vi "Dashboard Main.vi"() -> ()   [LabVIEW 2013]
uses:
  <vilib>/event_ctls.llb/eventvkey.ctl
  <vilib>/Rock Robotics/WPI/Dashboard/WPI_DashboardLogging Global.vi
  <vilib>/Utility/config.llb/Write Key (String).vi
  <vilib>/Utility/config.llb/Write Key (I32).vi
  <vilib>/Utility/config.llb/NI_LVConfig.lvlib
panel:
  out "Image Message":string="Timeout in Camera Communications"
  in  "Rec Mode":enum32{"Stop", "Record", "Playback"}(radio)
  in  "Dashboard Tab":T1(tab)=enum."Auto"
  in  "Camera Settings":T2={"Frame Rate"=30, "Compression"=30, "Size"=1} {"Frame Rate" scale=1.0..30.0; "Size" items=["640x480", "320x240", "160x120"]}
  out "MotorSliders R":cluster{"MotorSlide1":dbl, "MotorSlide2":dbl} {"MotorSlide2" scale=-1.0..1.0 scale format="%#_2e"; "MotorSlide1" scale=-1.0..1.0 scale format="%#_2e"}
  out "MotorChart R":cluster{"Numeric":dbl, "Numeric":dbl}(graph)
  out "MotorSliders L":T3 {"MotorSlide4 2" scale=0.0..14.0 scale format="%#_2e"; "MotorSlide2" scale=-1.0..1.0 scale format="%#_2e"; "MotorSlide1" scale=-1.0..1.0 scale format="%#_2e"}
  out "MotorChart L":T4(graph)
  out "JS1 Z":dbl(slide) scale=-1.0..1.0 scale format="%#_2e"
  out "Joystick 1":cluster{"X":dbl, "Y":dbl}[](graph)
  out "JS Buttons 1":T5
  out "JS2 Z":dbl(slide) scale=-1.0..1.0 scale format="%#_2e"
  out "Joystick 2":cluster{"X":dbl, "Y":dbl}[](graph)
  out "JS Buttons 2":T5
  out "Mode":T6(ring)=enum."Auto Disabled"
  out "Camera IP":string
  in  "DB Camera Config":bool
  out "fps":dbl format="%#.1g"
  out "Mbps":dbl format="%#.1g"
  out "Mbps 2":bool
  out "LED 1":bool
  in  "Slider 1":dbl(slide) scale=0.0..100.0
  in  "Auton Selection":dbl=5.0
  out "key":T7(ring)
  in  "Checkbox 2":bool
  in  "Checkbox 1":bool
  out "Code":dbl
  in  "Test Slider":dbl(slide) scale=0.0..100.0 scale format="%#_3g"
  in  "On/Off":bool caption="Solenoid"
  in  "Test Name":u16(ring) items=["Select the test to run...", "Example Test", "-------------------------------", "List of tests is built in robot code.", "Replace with your own automated tests."]
  in  "Test Tree":string(tree)
  in  "Motor":cluster{"Value":dbl, "Enable":bool} {"Value" scale=-1.0..1.0 scale format="%#_3g"}
  out "Progress":T8 {"Test Progress" scale=0.0..100.0}
  in  "Rev/Fwd":cluster{"Forward":bool, "Reverse":bool}
  in  "Test Ring":u16(ring) items=["Auto", "Fixed indoor", "Fixed outdoor 1", "Fixed outdoor 2", "Fixed fluorescent 1", "Fixed fluorescent 2", "Hold current"]
  in  "Listbox":i32(listbox)
  out "Tree":string(tree)
  out "Camera Image":T9(plugin-control)
  in  "Enable":bool
  # "Left"
  # "Front"
  # "Right"
  # "Battery"
  # "Customize by placing controls and indicators here and name to\nmatch Dashboard Variables on robot."
  # "This tab is a great place for autonomous settings and validation.\nCustomize by placing controls and indicators here and name to\nmatch Dashboard Variables on robot."
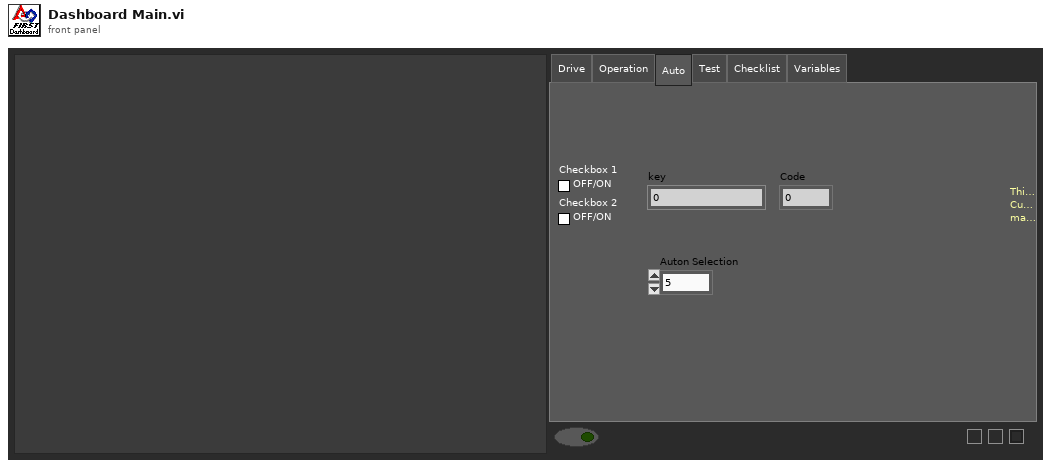
[diagram p1: front panel]
types:
  T1 = enum32{"Drive", "Operation", "Auto", "Test", "Checklist", "Variables"}
  T2 = cluster{"Frame Rate":i32, "Compression":i32, "Size":u16}
  T3 = cluster{"MotorSlide1":dbl, "MotorSlide2":dbl, "MotorSlide4 2":dbl}
  T4 = cluster{"Numeric":dbl, "Numeric":dbl, "Battery":sgl}
  T5 = cluster{bool, bool, bool, bool, bool, bool, bool, bool, bool, bool, bool, bool}
  T6 = enum8{"Tele-Op Disabled", "Tele-Op Enabled", "Auto Disabled", "Auto Enabled", "Test Disabled", "Test Enabled", ""}
  T7 = enum16{"0", "1", "2", "3", "4", "5", "6", "7", "8", "9", "A", "B", "C", "D", "E", "F", "G", "H", "I", "J", "K", "L", "M", "N", "O", "P", "Q", "R", "S", "T", "U", "V", "W", "X", "Y", "Z", "F1", "F2", "F3", "F4", "F5", "F6", "F7", "F8", "F9", "F10", "F11", "F12", "F13", "F14", "F15", "ADD", "BACK", "BACKSLASH", "CAPITAL", "COMMA", "DECIMAL", "DELETE", "DIVIDE", "DOWN", "END", "EQUALS", "ESCAPE", "GRAVE (`)", "HOME", "INSERT", "LBRACKET", "LCONTROL", "LEFT", "L ALT", "LSHIFT", "LWIN", "MINUS", "MULTIPLY", "NEXT", "NUMLOCK", "NUMPAD_0", "NUMPAD_1", "NUMPAD_2", "NUMPAD_3", "NUMPAD_4", "NUMPAD_5", "NUMPAD_6", "NUMPAD_7", "NUMPAD_8", "NUMPAD_9", "PAUSE", "PERIOD", "PRIOR (PG UP)", "RBRACKET", "RCONTROL", "RETURN", "RIGHT", "R ALT", "RSHIFT", "RWIN", "SCROLL", "SEMICOLON", "SLASH", "SPACE", "SUBTRACT", "TAB", "UP", "ENTER (num pad)", "' (quote)"}
  T8 = cluster{"Test Progress":u8, "Test Progress Text":string}
  T9 = typedef "IMAQ Image.ctl" = refnum<image>
  T10 = typedef "Image Type" = u32
  T11 = cluster{"Digital Inputs":bool[], "Digital Outputs":bool[]}
  T12 = cluster{"Competition mode":bool, "Robot Link":bool, "Autonomous":bool, "Enabled":bool, "E-Stop":bool, "Simulated":bool, "TestMode":bool, "Docked Window":bool}
  T13 = cluster{"Boolean Array[0]":bool, "Boolean Array[1]":bool, "Boolean Array[2]":bool, "Boolean Array[3]":bool, "Boolean Array[4]":bool, "Boolean Array[5]":bool, "Boolean Array[6]":bool, "Boolean Array[7]":bool, "Boolean Array[8]":bool, "Boolean Array[9]":bool, "Boolean Array[10]":bool, "Boolean Array[11]":bool}
  T14 = typedef "NI_LVConfig.lvlib/Config Data RefNum.ctl" = refnum<k1>
  T15 = typedef "eventvkey.ctl" = enum16{"ASCII", "Enter", "Return", "Shift", "Ctrl", "Alt", "Cmd", "Opt", "Caps", "NumLock", "Clear", "Break", "Up", "Down", "Left", "Right", "Insert", "Delete", "Home", "End", "PageUp", "PageDown", "Escape", "Help", "Pause", "ScrollLock", "F1", "F2", "F3", "F4", "F5", "F6", "F7", "F8", "F9", "F10", "F11", "F12", "F13", "F14", "F15", "F16", "F17", "F18", "F19", "F20", "F21", "F22", "F23", "F24", "Play", "VolumeUp", "VolumeDown", "Mute", "Two Byte Char"}
  T16 = cluster{"Image Size":bool, "Image Type":bool, "Pixel Value":bool, "ROI Information":bool, "Zoom Factor":bool}
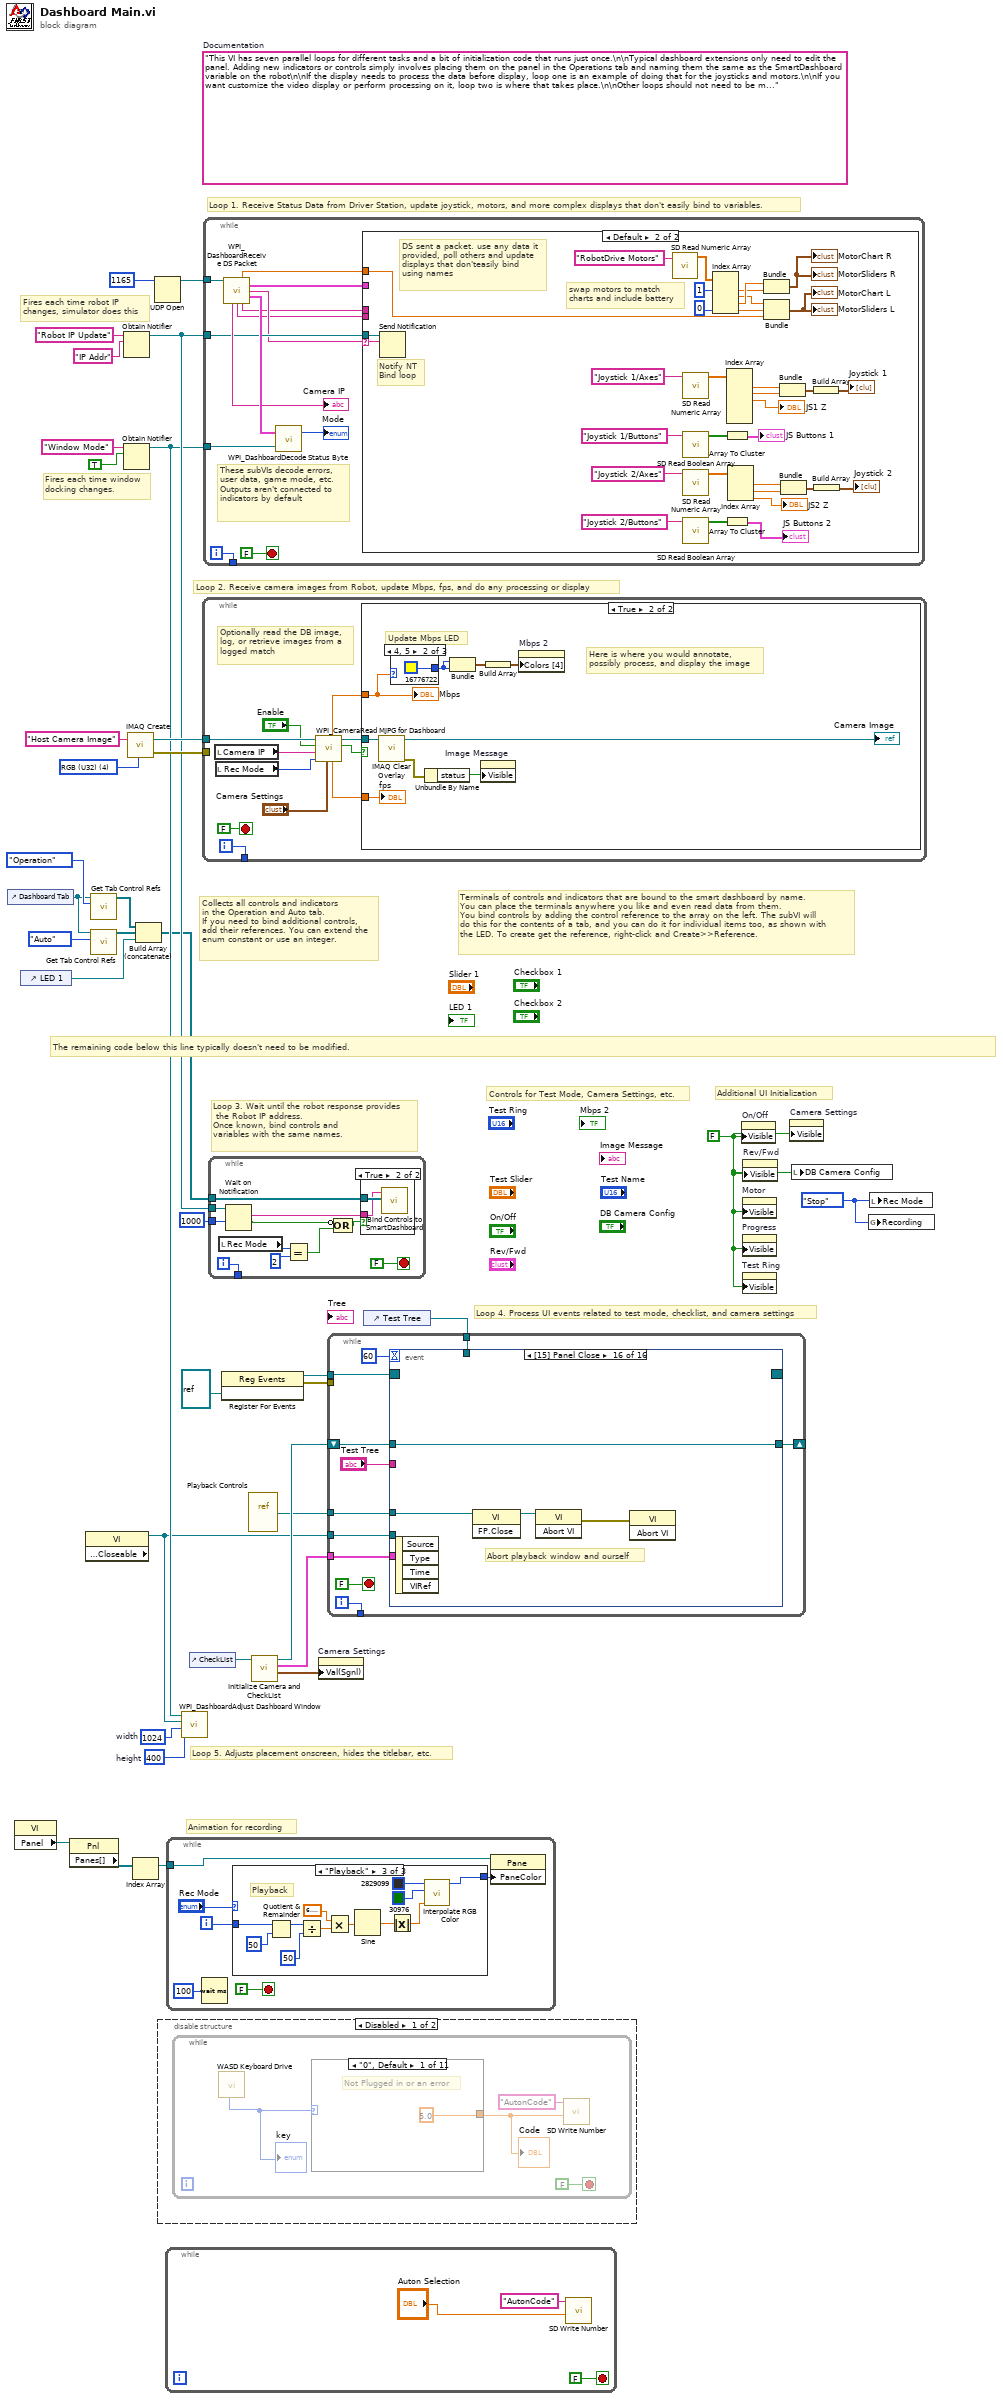
[diagram p0: block diagram]
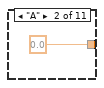
[diagram p2: hidden frame]
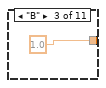
[diagram p3: hidden frame]
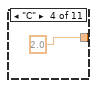
[diagram p4: hidden frame]
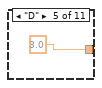
[diagram p5: hidden frame]
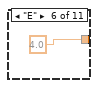
[diagram p6: hidden frame]
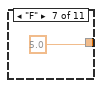
[diagram p7: hidden frame]
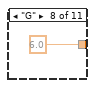
[diagram p8: hidden frame]
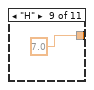
[diagram p9: hidden frame]
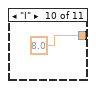
[diagram p10: hidden frame]
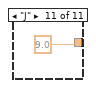
[diagram p11: hidden frame]
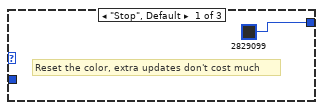
[diagram p13: hidden frame]
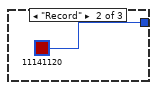
[diagram p14: hidden frame]
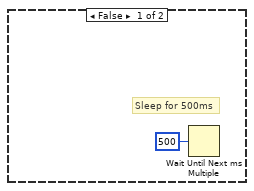
[diagram p16: hidden frame]
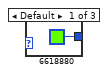
[diagram p17: hidden frame]
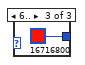
[diagram p18: hidden frame]
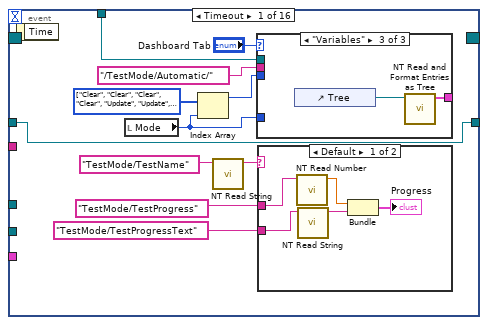
[diagram p19: hidden frame]
diagram:
  w8 = enum32{"Stop", "Record", "Playback"}."Stop" ("Rec Mode")
  w11 = 400  # height
  w12 = 1024  # width
  w25 = FALSE ("Visible")
  (unwired) "This VI has seven parallel loops for different tasks and a bit of initialization code that runs just once.\n\nTypical dashboard extensions only need to edit the panel. Adding new indicators or controls simply involves placing them on the panel in the Operations tab and naming them the same as the SmartDashboard variable on the robot\n\nIf the display needs to process the data before display, loop one is an example of doing that for the joysticks and motors.\n\nIf you want customize the video display or perform processing on it, loop two is where that takes place.\n\nOther loops should not need to be modified. They are pretty standard, and document the task they perform."  # Documentation
  w35 = T10 4 items=["Grayscale (U8)", "Grayscale (I16)", "Grayscale (SGL)", "Complex (CSG)", "RGB (U32)", "HSL (U32)", "RGB (U64)"] ("Image Type")
  # "Controls for Test Mode, Camera Settings, etc."
  # "Additional UI Initialization"
  # "Animation for recording"
  # "Fires each time robot IP\nchanges, simulator does this"
  # "Fires each time window\ndocking changes."
  # "Collects all controls and indicators\nin the Operation and Auto tab.\nIf you need to bind additional controls,\nadd their references. You can extend the\nenum constant or use an integer."
  # "The remaining code below this line typically doesn't need to be modified."
  # "Loop 4. Process UI events related to test mode, checklist, and camera settings"
  # "Terminals of controls and indicators that are bound to the smart dashboard by name.\nYou can place the terminals anywhere you like and even read data from them.\nYou bind controls by adding the control reference to the array on the left. The subVI will\ndo this for the contents of a tab, and you can do it for individual items too, as shown with\nthe LED. To create get the reference, right-click and Create>>Reference."
  # "Loop 3. Wait until the robot response provides\n the Robot IP address.\nOnce known, bind controls and\nvariables with the same names."
  # "Loop 5. Adjusts placement onscreen, hides the titlebar, etc."
  # "Loop 1. Receive Status Data from Driver Station, update joystick, motors, and more complex displays that don't easily bind to variables."
  # "Loop 2. Receive camera images from Robot, update Mbps, fps, and do any processing or display"
  n1 = control-ref of="Dashboard Tab"() -> (w6:refnum<vi>)
  n2 = property class="VI"() -> ("Panel"=w19:refnum<vi>)  [unwired: 2 in, 2 out]
  n3 = control-ref of="LED 1"() -> (w1:refnum<vi>)
  n4 = property class="Pnl"(reference=w19) -> ("Panes[]"=w20:refnum<vi>[])  [unwired: 1 in, 2 out]
  n5 = property class="VI" props=["Front Panel.Closeable"]() -> (reference out=w7:refnum<vi>)  [unwired: 2 in, 2 out]
  n6 = call <vilib>:"Get Tab Control Refs.vi"("Page Index"=T1."Operation" ("Dashboard Tab"), "TabControl in"=w6) -> ("ControlsOnPage"=w4:refnum<vi>[])  [unwired: 9 in]
  n7 = call <vilib>:"Get Tab Control Refs.vi"("Page Index"=T1."Auto" ("Dashboard Tab"), "TabControl in"=w6) -> ("ControlsOnPage"=w5:refnum<vi>[])  [unwired: 9 in]
  n8 = Obtain Notifier(name (unnamed)="Robot IP Update", notification data type="IP Addr" ("name (unnamed)")) -> (notifier out=w29:refnum<notifier>)  [unwired: 2 in, 2 out]
  n9 = Obtain Notifier(name (unnamed)="Window Mode", notification data type=TRUE) -> (notifier out=w10:refnum<notifier>)  [unwired: 2 in, 2 out]
  n10 = call "IMAQ Create"("Image Name"="Host Camera Image", "Image Type"=w35) -> ("New Image"=w33:T9, "error out"=w32:errorcluster)  [unwired: 2 in, 1 out]
  n11 = Index Array(array=w20) -> (element=w18:refnum<vi>)  [unwired: 1 in]
  n12 = Build Array (concatenate)(w4, w5, w1) -> (w3:refnum<vi>[])
  n13 = UDP Open(11:u16 1165 ("port")) -> (port=w36:refnum<k16>)  [unwired: 2 in, 4 out]
  n14 = disable-structure shown="Disabled" {
    frame Disabled {
      n15 = while {
        stop <- FALSE stop-if-true
        n16 = call "WASD Keyboard Drive.vi"() -> ("key"=w38:T7)  [unwired: 5 in, 2 out]
        "key" <- w38
        n17 = case shown="\"0\", Default" w38 {
          tunnel: [5.0 ("x") 0.0 ("x") 1.0 ("x") 2.0 ("x") 3.0 ("x") 4.0 ("x") 5.0 ("x") 6.0 ("x") 7.0 ("x") 8.0 ("x") 9.0 ("x")] -> w41
          frame "0", Default {
            # "Not Plugged in or an error"
          }
          frame "A" {
          }
          frame "B" {
          }
          frame "C" {
          }
          frame "D" {
          }
          frame "E" {
          }
          frame "F" {
          }
          frame "G" {
          }
          frame "H" {
          }
          frame "I" {
          }
          frame "J" {
          }
        }
        "Code" <- w41
        n18 = call <vilib>:"SD Write Number.vi"("Numeric"=w41, "Name"="AutonCode") -> ()  [unwired: 8 in, 2 out]
      }
    }
    frame Enabled {
    }
  }
  n19 = while {
    stop <- FALSE stop-if-true
    n20 = call <vilib>:"SD Write Number.vi"("Numeric"="Auton Selection", "Name"="AutonCode") -> ()  [unwired: 8 in, 2 out]
  }
  n21 = while {
    tunnel: w18 -> [w57]
    i -> [w60]
    stop <- FALSE stop-if-true
    n22 = Wait (ms)(milliseconds to wait=u32 100) -> ()  [unwired: 1 out]
    n23 = case shown="\"Playback\"" "Rec Mode" {
      tunnel: w60 -> [_ _ w75]
      tunnel: [u32 2829099 ("Base Color") u32 11141120 ("Target Color") w64] -> w56
      frame "Stop", Default {
        # "Reset the color, extra updates don't cost much"
      }
      frame "Record" {
      }
      frame "Playback" {
        # "Playback"
        n24 = Quotient & Remainder(x=w75, y=u32 50 ("milliseconds to wait")) -> (x-y*floor(x/y)=w71:u32)  [unwired: 1 out]
        n25 = Divide(x=w71, y=u32 50 ("milliseconds to wait")) -> (x/y=w68:dbl)
        n26 = Multiply(x=6.283185307179586, y=w68) -> (x*y=w73:dbl)
        n27 = Sine(x=w73) -> (sin(x)=w72:dbl)
        n28 = Absolute Value(x=w72) -> (abs(x)=w65:dbl)
        n29 = call "Interpolate RGB Color.vi"("Proportion"=w65, "Target Color"=u32 30976, "Base Color"=u32 2829099) -> ("Result Color"=w64:u32)  [unwired: 8 in]
      }
    }
    n30 = property class="Pane"(reference=w57, "PaneColor"=w56) -> ()  [unwired: 1 in, 2 out]
  }
  n31 = call <vilib>:"WPI_DashboardAdjust Dashboard Window.vi"("height"=w11, "width"=w12, "reference in"=w7, "Notifier in"=w10) -> ()  [unwired: 8 in]
  n32 = control-ref of="CheckList"() -> (w9:refnum<vi>)
  n33 = while {
    tunnel: w33 -> [w84]
    tunnel: w32 -> [_]
    tunnel: [w85] -> _
    i -> [w85]
    stop <- FALSE stop-if-true
    # "Optionally read the DB image,\nlog, or retrieve images from a\nlogged match"
    n34 = local read "Camera IP"() -> (w77:string)
    n35 = local read "Rec Mode"() -> (w76:enum32{"Stop", "Record", "Playback"})
    n36 = call <vilib>:"WPI_CameraRead MJPG for Dashboard.vi"("Camera Settings"="Camera Settings", "Rec Mode"=w76, "Camera IP"=w77, "Enable"="Enable", "Refnum in"=w84) -> ("Active"=w81:bool, "Refnum out"=w83:T9, "FPS"=w80:dbl, "Bandwidth (Mbps)"=w79:dbl)  [unwired: 3 in]
    n37 = case shown="True" w81 {
      tunnel: w83 -> [_ w91]
      tunnel: w79 -> [_ w90]
      tunnel: w80 -> [_ w88]
      frame False {
        # "Sleep for 500ms"
        n38 = Wait Until Next ms Multiple(millisecond multiple=u32 500) -> ()  [unwired: 1 out]
      }
      frame True {
        # "Here is where you would annotate,\npossibly process, and display the image"
        # "Update Mbps LED"
        n39 = call "IMAQ Clear Overlay"("Image"=w91) -> ("error out"=w95:errorcluster, "Image Out"=→"Camera Image":T9)  [unwired: 2 in, 7 out]
        n40 = case shown="4, 5" w90 {
          tunnel: [u32 6618880 ("Color Box") u32 16776722 ("Color Box") u32 16716800 ("Color Box")] -> w92
          frame Default {
          }
          frame 4, 5 {
          }
          frame 6.. {
          }
        }
        n41 = Unbundle By Name(w95) -> ("status"=w96:bool)
        n42 = Bundle("Color Box"=w92, "Color Box"=w92) -> (w94:cluster{"Color Box":u32, "Color Box":u32})  [unwired: 1 out]
        n43 = property on="Image Message" class="Str"("Visible"=w96) -> ()  [unwired: 2 in, 2 out]
        n44 = Build Array(w94) -> (w93:cluster{"Color Box":u32, "Color Box":u32}[])
        n45 = property on="Mbps 2" class="Bool (strict)"("Colors [4]"=w93) -> ()  [unwired: 2 in, 2 out]
        "Mbps" <- w90
        "fps" <- w88
      }
    }
  }
  n46 = while {
    tunnel: w36 -> [w110]
    tunnel: w29 -> [w105]
    tunnel: w10 -> [w109]
    tunnel: [w106] -> _
    i -> [w106]
    stop <- FALSE stop-if-true
    # "These subVIs decode errors, user data, game mode, etc.\nOutputs aren't connected to indicators by default"
    n47 = call <vilib>:"WPI_DashboardReceive DS Packet.vi"("Recv Socket"=w110) -> ("Battery"=w100:sgl, "Driver Station"=w101:T11, "Robot IP Address"=w104:string, "Status"=w111:T12, "Camera IP Address"=→"Camera IP":string, "Low Priority User Data"=w103:string, "High Priority User Data"=w102:string)  [unwired: 1 in, 7 out]
    n48 = call <vilib>:"WPI_DashboardDecode Status Byte.vi"("Window Mode Notifier"=w109, "Status"=w111) -> ("Mode"=→"Mode":T6)  [unwired: 1 out]
    n49 = case shown="Default" w104 {
      selector: w104 -> [_ w123]
      tunnel: w105 -> [_ w124]
      tunnel: w103 -> [_ _]
      tunnel: w102 -> [_ _]
      tunnel: w101 -> [_ _]
      tunnel: w100 -> [_ w122]
      frame "0.0.0.0" {
        # "DS not sending packets, or no robot exists yet.\nDon't poll the variables"
      }
      frame Default {
        # "Notify NT\nBind loop"
        # "DS sent a packet. use any data it\nprovided, poll others and update\ndisplays that don'teasily bind\nusing names"
        # "swap motors to match\ncharts and include battery"
        n50 = Send Notification(notification=w123, notifier=w124) -> ()  [unwired: 1 in, 2 out]
        n51 = call <vilib>:"SD Read Numeric Array.vi"("Name"="RobotDrive Motors") -> ("Numeric Array"=w121:dbl[])  [unwired: 8 in, 2 out]
        n52 = call <vilib>:"SD Read Numeric Array.vi"("Name"="Joystick 1/Axes") -> ("Numeric Array"=w140:dbl[])  [unwired: 8 in, 2 out]
        n53 = call <vilib>:"SD Read Boolean Array.vi"("Name"="Joystick 1/Buttons") -> ("Boolean Array"=w142:bool[])  [unwired: 8 in, 2 out]
        n54 = call <vilib>:"SD Read Numeric Array.vi"("Name"="Joystick 2/Axes") -> ("Numeric Array"=w134:dbl[])  [unwired: 8 in, 2 out]
        n55 = call <vilib>:"SD Read Boolean Array.vi"("Name"="Joystick 2/Buttons") -> ("Boolean Array"=w133:bool[])  [unwired: 8 in, 2 out]
        n56 = Index Array(array=w121, index #1=1, index #4=0) -> (element #1=w117:dbl, element #2=w116:dbl, element #3=w118:dbl, element #4=w113:dbl)  [unwired: 2 in]
        n57 = Array To Cluster(array=w142) -> (cluster=→"JS Buttons 1":T13)
        n58 = Array To Cluster(array=w133) -> (cluster=→"JS Buttons 2":T13)
        n59 = Index Array(array=w140) -> (element #1=w137:dbl, element #2=w138:dbl, element #3=→"JS1 Z":dbl)  [unwired: 6 in, 3 out]
        n60 = Index Array(array=w134) -> (element #1=w129:dbl, element #2=w128:dbl, element #3=→"JS2 Z":dbl)  [unwired: 3 in]
        n61 = Bundle("Numeric"=w118, "Numeric"=w117) -> (→"MotorChart R" →"MotorSliders R":cluster{"Numeric":dbl, "Numeric":dbl})  [unwired: 1 in]
        n62 = Bundle("Numeric"=w116, "Numeric"=w113, "Battery"=w122) -> (→"MotorChart L" →"MotorSliders L":T4)  [unwired: 1 in]
        n63 = Bundle("Numeric"=w137, "Numeric"=w138) -> (w136:cluster{"Numeric":dbl, "Numeric":dbl})  [unwired: 1 in]
        n64 = Bundle("Numeric"=w129, "Numeric"=w128) -> (w130:cluster{"Numeric":dbl, "Numeric":dbl})  [unwired: 1 in]
        n65 = Build Array(w136) -> (→"Joystick 1":cluster{"Numeric":dbl, "Numeric":dbl}[])
        n66 = Build Array(w130) -> (→"Joystick 2":cluster{"Numeric":dbl, "Numeric":dbl}[])
      }
    }
  }
  n67 = while {
    tunnel: w3 -> [w156]
    tunnel: w29 -> [w154]
    tunnel: [w152] -> _
    tunnel: u32 1000 ("milliseconds to wait") -> [w151]
    i -> [w152]
    stop <- FALSE stop-if-true
    n68 = local read "Rec Mode"() -> (w147:enum32{"Stop", "Record", "Playback"})
    n69 = Wait on Notification(notifier=w154, timeout in ms (-1)=w151) -> (notification=w153:string, timed out?=w149:bool)  [unwired: 2 in, 2 out]
    n70 = Equal?(x=w147, y=u16 2 ("Rec Mode")) -> (x = y?=w148:bool)
    n71 = Compound Arithmetic op=OR(invert w149, w148) -> (w150:bool)
    n72 = case shown="True" w150 {
      tunnel: w156 -> [_ w158]
      tunnel: w153 -> [_ w157]
      frame False {
      }
      frame True {
        n73 = call <vilib>:"Bind Controls to SmartDashboard.vi"("Bound Control Refs"=w158, "Server IP Address"=w157) -> ()  [unwired: 10 in]
      }
    }
  }
  n74 = register-events(refnum<vi> refnum) -> (reference out=w16:refnum<event-registration>, error out=w15:errorcluster)  [unwired: 2 in]
  n75 = vi-ref "Playback Controls.vi"() -> (w17:refnum<vi>)
  n76 = call "Initialize Camera and CheckList.vi"("ListBox in"=w9) -> ("Cluster"=w23:cluster{"value":i32, "value":i32, "index":i32}, "Array"=w24:cluster{string[]}[], "File Refnum"=w22:T14)  [unwired: 8 in]
  n77 = property on="Camera Settings" class="Clust (strict)"("Val(Sgnl)"=w23) -> ()  [unwired: 2 in, 2 out]
  n78 = control-ref of="Test Tree"() -> (w21:refnum<vi>)
  n79 = while {
    tunnel: w24 -> [w166]
    shift-right: [w165] -> _
    shift-left: w22 -> [w164]
    tunnel: [w163] -> _
    tunnel: w21 -> [w162]
    tunnel: w17 -> [w161]
    tunnel: w16 -> [w160]
    tunnel: w15 -> [_]
    tunnel: w7 -> [w159]
    i -> [w163]
    stop <- FALSE stop-if-true
    n80 = event shown="[15] Panel Close" {
      selector: w160 -> [_ _ _ _ _ _ _ _ _ _ _ _ _ _ _ _]
      dyn-events: [_ _ _ _ _ _ _ _ _ _ _ _ _ w404 _ _] -> _
      timeout: u32 60 ("milliseconds to wait") -> [_ _ _ _ _ _ _ _ _ _ _ _ _ _ _ _]
      tunnel: w162 -> [w176 _ _ _ _ _ _ _ _ _ _ _ _ _ _ _]
      tunnel: "Test Tree" -> [_ _ _ _ _ _ _ _ w373 w381 w383 w387 w395 _ _ _]
      tunnel: w166 -> [_ w200 _ _ _ _ w337 w367 _ _ _ _ _ _ _ _]
      tunnel: [w170 w199 w298 w303 w311 w323 w336 w360 w372 w379 w382 w386 w394 w406 w420 w421] -> w165
      tunnel: w164 -> [w170 w199 w298 w303 w311 w323 w335 w360 w372 w379 w382 w386 w394 w406 w420 w421]
      tunnel: w161 -> [_ _ _ _ _ _ _ _ _ _ _ _ _ w407 _ w424]
      tunnel: w159 -> [_ _ _ _ _ _ _ _ _ _ _ _ _ w402 _ _]
      event Timeout {
        w175 = enum16{"Update", "Clear"}[] [enum."Clear", enum."Clear", enum."Clear", enum."Clear", enum."Update", enum."Update", enum."Clear"] items=["Update", "Clear"]
        n81 = event-data() -> ()  [unwired: 1 in, 1 out]
        n82 = local read "Mode"() -> (w173:T6)
        n83 = Index Array(array=w175, index=w173) -> (element=w174:enum16{"Update", "Clear"})
        n84 = call <vilib>:"NT Read String.vi"("Name"="TestMode/TestName") -> ("String"=w179:string)  [unwired: 9 in, 1 out]
        n85 = case shown="\"Variables\"" "Dashboard Tab" {
          tunnel: w176 -> [_ w189 _]
          tunnel: "/TestMode/Automatic/" ("Name Pattern") -> [_ w188 _]
          tunnel: w174 -> [_ w187 _]
          tunnel: w173 -> [_ w185 _]
          tunnel: [_ _ w191] -> _
          frame "Operation", Default {
          }
          frame "Test" {
            w184 = -2 ("Active Item:Row Number")
            n86 = call <vilib>:"NT Read and Format Entries as Tree.vi"("Operation"=w187, "Name Pattern"=w188, "Tree Refnum"=w189) -> ()  [unwired: 7 in, 2 out]
            n87 = Index Array(array=u32[] [14013909, 14013909, 14013909, 14013909, 14013909, 16777215, 14013909], index=w185) -> (element=w183:u32)
            n88 = property on="Test Tree" class="Tree (strict)"("Active Item Row Number"=w184, "ActiveColNum"=w184, "CellBG"=w183, "Active Item Row Number"=-1 ("Active Item:Row Number"), "CellBG"=u32 5789784 ("Color Box")) -> ()  [unwired: 2 in, 2 out]
          }
          frame "Variables" {
            n89 = control-ref of="Tree"() -> (w190:refnum<vi>)
            n90 = call <vilib>:"NT Read and Format Entries as Tree.vi"("Tree Refnum"=w190) -> ("Formatted Strings"=w191:cluster{"Name":string, "Value":string}[])  [unwired: 9 in, 1 out]
          }
        }
        n91 = case shown="Default" w179 {
          tunnel: "TestMode/TestProgress" ("Name") -> [w193 _]
          tunnel: "TestMode/TestProgressText" ("Name") -> [w192 _]
          frame Default {
            n92 = call <vilib>:"NT Read Number.vi"("Name"=w193) -> ("Numeric"=w194:dbl)  [unwired: 9 in, 1 out]
            n93 = call <vilib>:"NT Read String.vi"("Name"=w192) -> ("String"=w195:string)  [unwired: 9 in, 1 out]
            n94 = Bundle("Numeric"=w194, "String"=w195) -> (→"Progress":cluster{"Numeric":dbl, "String":string})  [unwired: 1 in]
          }
          frame "" {
            n95 = property on="Progress" class="Clust (strict)"("Visible"=FALSE) -> ()  [unwired: 2 in, 2 out]
            n96 = local write "Test Name"(u16 0) -> ()
          }
        }
      }
      event "Test Tree": Value Change {
        # "Show appropriate\ncontrols"
        n97 = event-data() -> ("CtlRef"=w203:refnum<vi>, "NewVal"=w201:string)  [unwired: 1 in]
        n98 = call <vilib>:"WPI_UtilitiesGetTreeIOName.vi"("NewVal"=w201, "TreeControl in"=w203) -> ("I/O Name"=w204:string)  [unwired: 9 in]
        n99 = case shown="\"Camera\"" w204 {
          selector: w204 -> [_ w211 _ w229 w238 _]
          tunnel: w201 -> [_ _ w226 w228 _ w245]
          tunnel: w200 -> [_ _ _ _ _ w244]
          frame Default {
            w206 = FALSE ("Visible")
            w205 = FALSE ("Visible")
            n100 = property on="Motor" class="Clust (strict)"("Visible"=w205) -> ()  [unwired: 2 in, 2 out]
            n101 = property on="Test Ring" class="Ring (strict)"("Visible"=w205) -> ()  [unwired: 2 in, 2 out]
            n102 = property on="Rev/Fwd" class="Clust (strict)"("Visible"=w206) -> ()  [unwired: 2 in, 2 out]
            n103 = property on="On/Off" class="Bool (strict)"("Visible"=w206) -> ()  [unwired: 2 in, 2 out]
            n104 = property on="Test Slider" class="Slide (strict)"("Visible"=w206) -> ()  [unwired: 2 in, 2 out]
          }
          frame "Motor", "PWM" {
            w212 = FALSE ("Visible")
            n105 = case shown="\"Motor\", Default" w211 {
              tunnel: [1.0 ("Value") -1.0 ("Value")] -> w210
              tunnel: [255.0 ("Value") 1.0 ("Value")] -> w209
              tunnel: [128.0 ("Value") 0.0 ("Value")] -> w208
              tunnel: [64.0 ("Value") 0.5 ("Value")] -> w207
              frame "PWM" {
              }
              frame "Motor", Default {
              }
            }
            n106 = property on="Motor" class="Clust (strict)"("Visible"=TRUE) -> ()  [unwired: 2 in, 2 out]
            n107 = property on="Value" class="Slide (strict)"("Value"=w208, "Scale.Minimum"=w210, "Scale.Maximum"=w209, "Scale.Increment"=w207) -> ()  [unwired: 2 in, 2 out]
            n108 = property on="On/Off" class="Bool (strict)"("Visible"=w212) -> ()  [unwired: 2 in, 2 out]
            n109 = property on="Test Slider" class="Slide (strict)"("Visible"=w212) -> ()  [unwired: 2 in, 2 out]
            n110 = property on="Test Ring" class="Ring (strict)"("Visible"=w212) -> ()  [unwired: 2 in, 2 out]
            n111 = property on="Rev/Fwd" class="Clust (strict)"("Visible"=w212) -> ()  [unwired: 2 in, 2 out]
          }
          frame "Servo" {
            w224 = FALSE ("Visible")
            n112 = call <vilib>:"NT Read Number.vi"("Name"=w226) -> ("Numeric"=w225:dbl)  [unwired: 9 in, 1 out]
            n113 = property on="Test Slider" class="Slide (strict)"("Visible"=TRUE, "Scale.Maximum"=170.0 ("Scale.Range:Maximum")) -> ()  [unwired: 2 in, 2 out]
            n114 = local write "Test Slider"(w225) -> ()
            n115 = property on="Motor" class="Clust (strict)"("Visible"=w224) -> ()  [unwired: 2 in, 2 out]
            n116 = property on="Rev/Fwd" class="Clust (strict)"("Visible"=w224) -> ()  [unwired: 2 in, 2 out]
            n117 = property on="On/Off" class="Bool (strict)"("Visible"=w224) -> ()  [unwired: 2 in, 2 out]
            n118 = property on="Test Ring" class="Ring (strict)"("Visible"=w224) -> ()  [unwired: 2 in, 2 out]
          }
          frame "Relay", "Solenoid" {
            w227 = FALSE ("Visible")
            n119 = property on="Motor" class="Clust (strict)"("Visible"=w227) -> ()  [unwired: 2 in, 2 out]
            n120 = property on="Test Slider" class="Slide (strict)"("Visible"=w227) -> ()  [unwired: 2 in, 2 out]
            n121 = Search and Replace String(input string=w228, search string="/Value  **", replace string="/Direction") -> (result string=w234:string)  [unwired: 5 in, 3 out]
            n122 = property on="Test Ring" class="Ring (strict)"("Visible"=w227) -> ()  [unwired: 2 in, 2 out]
            n123 = call <vilib>:"NT Read String.vi"("Name"=w234) -> ("String"=w232:string)  [unwired: 9 in, 1 out]
            n124 = Equal?(x="Both directions", y=w232) -> (x = y?=w230:bool)
            n125 = Not(x=w230) -> (.not. x?=w231:bool)
            n126 = property on="Rev/Fwd" class="Clust (strict)"("Visible"=w230) -> ()  [unwired: 2 in, 2 out]
            n127 = property on="On/Off" class="Bool (strict)"("Visible"=w231, "Caption.Text"=w229) -> ()  [unwired: 2 in, 2 out]
          }
          frame "Compressor", "Digital Out" {
            w237 = FALSE ("Visible")
            # "Get direction and finish"
            n128 = property on="Motor" class="Clust (strict)"("Visible"=w237) -> ()  [unwired: 2 in, 2 out]
            n129 = property on="Test Slider" class="Slide (strict)"("Visible"=w237) -> ()  [unwired: 2 in, 2 out]
            n130 = property on="Test Ring" class="Ring (strict)"("Visible"=w237) -> ()  [unwired: 2 in, 2 out]
            n131 = property on="On/Off" class="Bool (strict)"("Visible"=TRUE, "Caption.Text"=w238) -> ()  [unwired: 2 in, 2 out]
            n132 = property on="Rev/Fwd" class="Clust (strict)"("Visible"=FALSE) -> ()  [unwired: 2 in, 2 out]
          }
          frame "Camera" {
            n133 = call <vilib>:"Get Last Path Segment.vi"("String in"=w245) -> ("String out"=w246:string)  [unwired: 10 in]
            n134 = property on="On/Off" class="Bool (strict)"("Visible"=FALSE) -> ()  [unwired: 2 in, 2 out]
            n135 = property on="Motor" class="Clust (strict)"("Visible"=FALSE) -> ()  [unwired: 2 in, 2 out]
            n136 = property on="Rev/Fwd" class="Clust (strict)"("Visible"=FALSE) -> ()  [unwired: 2 in, 2 out]
            n137 = case shown="\"White Balance  **\"" w246 {
              tunnel: w245 -> [w252 w261 w270 w279 w288 _ w294]
              tunnel: w244 -> [w250 w258 w267 w276 w285 _ _]
              frame "Size  **" {
                n138 = Index Array(array=w250) -> (element=w249:cluster{string[]})  [unwired: 1 in]
                n139 = call <vilib>:"NT Read String.vi"("Name"=w252) -> ("String"=w251:string)  [unwired: 9 in, 1 out]
                n140 = Unbundle(w249) -> (w247:string[])
                n141 = Match First String(2:w247, 3:w251) -> (0:w248:i32)  [unwired: 1 out]
                n142 = property on="Test Ring" class="Ring (strict)"("Value"=w248, "Strings []"=w247) -> ()  [unwired: 2 in, 2 out]
                n143 = property on="Test Ring" class="Ring (strict)"("Visible"=TRUE) -> ()  [unwired: 2 in, 2 out]
                n144 = property on="Test Slider" class="Slide (strict)"("Visible"=FALSE) -> ()  [unwired: 2 in, 2 out]
              }
              frame "White Balance  **" {
                n145 = Index Array(array=w258, index=1) -> (element=w259:cluster{string[]})
                n146 = call <vilib>:"NT Read String.vi"("Name"=w261) -> ("String"=w260:string)  [unwired: 9 in, 1 out]
                n147 = Unbundle(w259) -> (w256:string[])
                n148 = Match First String(2:w256, 3:w260) -> (0:w255:i32)  [unwired: 1 out]
                n149 = property on="Test Ring" class="Ring (strict)"("Value"=w255, "Strings []"=w256) -> ()  [unwired: 2 in, 2 out]
                n150 = property on="Test Ring" class="Ring (strict)"("Visible"=TRUE) -> ()  [unwired: 2 in, 2 out]
                n151 = property on="Test Slider" class="Slide (strict)"("Visible"=FALSE) -> ()  [unwired: 2 in, 2 out]
              }
              frame "Exposure  **" {
                n152 = Index Array(array=w267, index=2) -> (element=w268:cluster{string[]})
                n153 = call <vilib>:"NT Read String.vi"("Name"=w270) -> ("String"=w269:string)  [unwired: 9 in, 1 out]
                n154 = Unbundle(w268) -> (w264:string[])
                n155 = Match First String(2:w264, 3:w269) -> (0:w265:i32)  [unwired: 1 out]
                n156 = property on="Test Ring" class="Ring (strict)"("Value"=w265, "Strings []"=w264) -> ()  [unwired: 2 in, 2 out]
                n157 = property on="Test Ring" class="Ring (strict)"("Visible"=TRUE) -> ()  [unwired: 2 in, 2 out]
                n158 = property on="Test Slider" class="Slide (strict)"("Visible"=FALSE) -> ()  [unwired: 2 in, 2 out]
              }
              frame "Exposure Priority  **" {
                n159 = Index Array(array=w276, index=3) -> (element=w277:cluster{string[]})
                n160 = call <vilib>:"NT Read String.vi"("Name"=w279) -> ("String"=w278:string)  [unwired: 9 in, 1 out]
                n161 = Unbundle(w277) -> (w273:string[])
                n162 = Match First String(2:w273, 3:w278) -> (0:w274:i32)  [unwired: 1 out]
                n163 = property on="Test Ring" class="Ring (strict)"("Value"=w274, "Strings []"=w273) -> ()  [unwired: 2 in, 2 out]
                n164 = property on="Test Ring" class="Ring (strict)"("Visible"=TRUE) -> ()  [unwired: 2 in, 2 out]
                n165 = property on="Test Slider" class="Slide (strict)"("Visible"=FALSE) -> ()  [unwired: 2 in, 2 out]
              }
              frame "Color Enable  **" {
                n166 = Index Array(array=w285, index=4) -> (element=w286:cluster{string[]})
                n167 = call <vilib>:"NT Read String.vi"("Name"=w288) -> ("String"=w287:string)  [unwired: 9 in, 1 out]
                n168 = Unbundle(w286) -> (w282:string[])
                n169 = Match First String(2:w282, 3:w287) -> (0:w283:i32)  [unwired: 1 out]
                n170 = property on="Test Ring" class="Ring (strict)"("Value"=w283, "Strings []"=w282) -> ()  [unwired: 2 in, 2 out]
                n171 = property on="Test Ring" class="Ring (strict)"("Visible"=TRUE) -> ()  [unwired: 2 in, 2 out]
                n172 = property on="Test Slider" class="Slide (strict)"("Visible"=FALSE) -> ()  [unwired: 2 in, 2 out]
              }
              frame Default {
                n173 = property on="Test Ring" class="Ring (strict)"("Visible"=FALSE) -> ()  [unwired: 2 in, 2 out]
                n174 = property on="Test Slider" class="Slide (strict)"("Visible"=FALSE) -> ()  [unwired: 2 in, 2 out]
              }
              frame "Brightness  **", "Color Level  **", "Compression  **", "FPS  **", "Sharpness  **" {
                n175 = call <vilib>:"NT Read Number.vi"("Name"=w294) -> ("Numeric"=w293:dbl)  [unwired: 9 in, 1 out]
                n176 = local write "Test Slider"(w293) -> ()
                n177 = property on="Test Slider" class="Slide (strict)"("Visible"=TRUE, "Scale.Maximum"=100.0 ("Scale.Range:Maximum")) -> ()  [unwired: 2 in, 2 out]
                n178 = property on="Test Ring" class="Ring (strict)"("Visible"=FALSE) -> ()  [unwired: 2 in, 2 out]
              }
            }
          }
        }
        n179 = property on="Progress" class="Clust (strict)"("Visible"=FALSE) -> ()  [unwired: 2 in, 2 out]
      }
      event "Test Name": Mouse Enter {
        # "Populate the ring with the list of tests"
        n180 = event-data() -> ()  [unwired: 1 in, 1 out]
        n181 = call <vilib>:"NT Read String Array.vi"("Name"="TestMode/TestList") -> ("String Array"=w302:string[])  [unwired: 9 in, 1 out]
        n182 = Build Array (concatenate)("Select the test to run...", w302) -> (w301:string[])
        n183 = property on="Test Name" class="Ring (strict)"("Strings []"=w301) -> ()  [unwired: 2 in, 2 out]
      }
      event "Test Name": Value Change {
        w304 = FALSE ("Visible")
        # "Tell the robot the test name to run"
        n184 = event-data() -> ("NewVal"=w308:u16)  [unwired: 1 in]
        n185 = property on="Test Name" class="Ring (strict)"() -> ("Strings []"=w309:string[])  [unwired: 2 in, 2 out]
        n186 = local write "Progress"(T8 {"Test Progress"=0, "Test Progress Text"=""} ("Progress")) -> ()
        n187 = Index Array(array=w309, index=w308) -> (element=w307:string)
        n188 = call <vilib>:"NT Write String.vi"("String"=w307, "Name"="TestMode/TestName") -> ()  [unwired: 9 in, 1 out]
        n189 = property on="Progress" class="Clust (strict)"("Visible"=TRUE) -> ()  [unwired: 2 in, 2 out]
        n190 = property on="Motor" class="Clust (strict)"("Visible"=w304) -> ()  [unwired: 2 in, 2 out]
        n191 = property on="Test Slider" class="Slide (strict)"("Visible"=w304) -> ()  [unwired: 2 in, 2 out]
        n192 = property on="On/Off" class="Bool (strict)"("Visible"=w304) -> ()  [unwired: 2 in, 2 out]
        n193 = property on="Rev/Fwd" class="Clust (strict)"("Visible"=w304) -> ()  [unwired: 2 in, 2 out]
        n194 = property on="Test Ring" class="Ring (strict)"("Visible"=w304) -> ()  [unwired: 2 in, 2 out]
      }
      event "Listbox": Double Click {
        n195 = event-data() -> ("PlatMods.Shift"=w312:bool, "Row"=w314:i32)  [unwired: 1 in]
        n196 = case shown="True" w312 {
          tunnel: w314 -> [w318 _]
          tunnel: 1 -> [w317 _]
          frame False {
            n197 = property on="Listbox" class="LstBox (strict)"() -> ("Item Symbols"=w316:i32[])  [unwired: 2 in, 2 out]
            n198 = Replace Array Subset(array=w316, new element=w317, index=w318) -> (w315:i32[])
            n199 = property on="Listbox" class="LstBox (strict)"("Item Symbols"=w315) -> ()  [unwired: 2 in, 2 out]
          }
          frame True {
            w319 = 0 ("Top Row")
            n200 = property on="Listbox" class="LstBox (strict)"() -> ("Number of Rows"=w321:u32)  [unwired: 2 in, 2 out]
            n201 = Initialize Array(0, w321) -> (w320:i32[])
            n202 = property on="Listbox" class="LstBox (strict)"("Top Row"=w319, "Value"=w319, "Item Symbols"=w320) -> ()  [unwired: 2 in, 2 out]
          }
        }
      }
      event "Listbox": Key Down {
        n203 = event-data() -> ("VKey"=w325:T15)  [unwired: 1 in]
        n204 = case shown="\"Left\", \"Right\"" w325 {
          selector: w325 -> [w330 _]
          tunnel: eventvkey."Left" ("VKey") -> [w328 _]
          frame "Left", "Right" {
            n205 = Equal?(x=w328, y=w330) -> (x = y?=w329:bool)
            n206 = Select(t=0, s=w329, f=1) -> (s? t:f=w331:i32)
            n207 = property on="Listbox" class="LstBox (strict)"() -> ("Item Symbols"=w334:i32[])  [unwired: 2 in, 2 out]
            n208 = Replace Array Subset(array=w334, new element=w331, index="Listbox") -> (w333:i32[])
            n209 = property on="Listbox" class="LstBox (strict)"("Item Symbols"=w333) -> ()  [unwired: 2 in, 2 out]
          }
          frame Default {
          }
        }
      }
      event "DB Camera Config": Value Change {
        n210 = event-data() -> ("NewVal"=w338:bool)  [unwired: 1 in]
        n211 = case shown="False" w338 {
          tunnel: w337 -> [w347 _]
          tunnel: [w340 w358] -> w336
          tunnel: w335 -> [w339 w358]
          frame False {
            w354 = "Camera"
            w357 = FALSE ("Visible")
            n212 = local read "Camera Settings"() -> (w346:T2)
            n213 = Index Array(array=w347) -> (element=w350:cluster{string[]})  [unwired: 1 in]
            n214 = Unbundle(w346) -> ("Frame Rate"=w345:i32, "Compression"=w344:i32, "Size"=w348:u16)
            n215 = Unbundle(w350) -> (w349:string[])
            n216 = Index Array(array=w349, index=w348) -> (element=w343:string)
            n217 = call-poly <vilib>:"Write Key.vi"("section"=w354, "value"=w343, "key"="Size", "refnum"=w339) -> ("refnum out"=w356:T14)  [unwired: 2 in, 5 out]
            n218 = call-poly <vilib>:"Write Key.vi"("section"=w354, "value"=w345, "key"="FrameRate", "refnum"=w356) -> ("refnum out"=w355:T14)  [unwired: 1 in, 6 out]
            n219 = property on="Camera Settings" class="Clust (strict)"("Visible"=w357) -> ()  [unwired: 2 in, 2 out]
            n220 = local write "DB Camera Config"(w357) -> ()
            n221 = call-poly <vilib>:"Write Key.vi"("section"=w354, "value"=w344, "key"="Compression", "refnum"=w355) -> ("refnum out"=w341:T14)  [unwired: 1 in, 6 out]
            n222 = call <vilib>:"Close Config Data.vi"("refnum"=w341) -> ("file path"=w342:path)  [unwired: 2 in, 8 out]
            n223 = call <vilib>:"Open Config Data.vi"("configuration file path"=w342) -> ("refnum"=w340:T14)  [unwired: 8 in, 2 out]
          }
          frame True {
            n224 = property on="Camera Settings" class="Clust (strict)"("Visible"=TRUE) -> ()  [unwired: 2 in, 2 out]
          }
        }
      }
      event "Camera Settings": Value Change {
        n225 = event-data() -> ("NewVal"=w371:T2)  [unwired: 1 in]
        n226 = Index Array(array=w367) -> (element=w366:cluster{string[]})  [unwired: 1 in]
        n227 = Unbundle(w371) -> ("Frame Rate"=w362:i32, "Compression"=w361:i32, "Size"=w364:u16)
        n228 = Unbundle(w366) -> (w365:string[])
        n229 = Index Array(array=w365, index=w364) -> (element=w363:string)
        n230 = Format Into String(format string="%s   %dfps   %d%%", w363, w362, w361) -> (resulting string=w368:string)  [unwired: 2 in, 1 out]
        n231 = Build Array(w368) -> (w369:string[])
        n232 = property on="DB Camera Config" class="Bool (strict)"("Strings [4]"=w369) -> ()  [unwired: 2 in, 2 out]
      }
      event "Motor.Enable": Value Change {
        n233 = event-data() -> ("NewVal"=w377:bool)  [unwired: 1 in]
        n234 = Unbundle("Motor") -> ("Value"=w376:dbl)  [unwired: 1 out]
        n235 = Select(t=w376, s=w377, f=0.0) -> (s? t:f=w374:dbl)
        n236 = call <vilib>:"NT Write Number.vi"("Numeric"=w374, "Name"=w373) -> ()  [unwired: 9 in, 1 out]
      }
      event "Test Slider": Value Change {
        n237 = event-data() -> ("NewVal"=w380:dbl)  [unwired: 1 in]
        n238 = call <vilib>:"NT Write Number.vi"("Numeric"=w380, "Name"=w381) -> ()  [unwired: 9 in, 1 out]
      }
      event "On/Off": Value Change {
        n239 = event-data() -> ("NewVal"=w385:bool)  [unwired: 1 in]
        n240 = Boolean To (0,1)(Boolean=w385) -> (0, 1=w384:i16)
        n241 = call <vilib>:"NT Write Number.vi"("Numeric"=w384, "Name"=w383) -> ()  [unwired: 9 in, 1 out]
      }
      event "Rev/Fwd": Value Change {
        n242 = event-data() -> ("NewVal.Forward"=w393:bool, "NewVal.Reverse"=w392:bool)  [unwired: 1 in]
        n243 = Boolean To (0,1)(Boolean=w393) -> (0, 1=w389:i16)
        n244 = Boolean To (0,1)(Boolean=w392) -> (0, 1=w391:i16)
        n245 = Negate(x=w391) -> (-x=w390:i16)
        n246 = Add(x=w389, y=w390) -> (x+y=w388:i16)
        n247 = call <vilib>:"NT Write Number.vi"("Numeric"=w388, "Name"=w387) -> ()  [unwired: 9 in, 1 out]
      }
      event "Test Ring": Value Change {
        n248 = event-data() -> ("NewVal"=w397:u16)  [unwired: 1 in]
        n249 = property on="Test Ring" class="Ring (strict)"() -> ("Strings []"=w398:string[])  [unwired: 2 in, 2 out]
        n250 = Index Array(array=w398, index=w397) -> (element=w396:string)
        n251 = call <vilib>:"NT Write String.vi"("String"=w396, "Name"=w395) -> ()  [unwired: 9 in, 1 out]
      }
      event "Rec Mode": Value Change {
        # "Update globals for recording mode and path to read log from.\nClear when logging and let NetworkTables set path for vision to\nuse."
        n252 = event-data() -> ("NewVal"=w408:enum32{"Stop", "Record", "Playback"})  [unwired: 1 in]
        n253 = global write "WPI_DashboardLogging Global.vi" "Logging Filename"(path "") -> ()
        n254 = case shown="\"Stop\", \"Record\"" w408 {
          tunnel: w407 -> [_ w410 w418]
          tunnel: [_ _ w417] -> w404
          tunnel: [_ _ w416] -> _
          tunnel: w402 -> [_ _ w414]
          tunnel: cluster{i32, i32} {-250, 170} -> [_ _ w413]
          tunnel: [_ _ T16 {"Image Size"=TRUE, "Image Type"=TRUE, "Pixel Value"=TRUE, "ROI Information"=TRUE, "Zoom Factor"=FALSE} ("Image Information Shown:All Elements")] -> w400
          tunnel: [_ _ TRUE ("Zoom Factor")] -> w399
          frame Default {
          }
          frame "Stop", "Record" {
            # "Place Window too"
            n255 = invoke class="VI" method="FP.Close"(reference=w410) -> (reference out=w409:refnum<vi>)  [unwired: 2 in, 2 out]
            n256 = invoke class="VI" method="Abort VI"(reference=w409) -> ()  [unwired: 2 in, 3 out]
          }
          frame "Playback" {
            n257 = call "Open Playback Panel.vi"("Offset"=w413, "DB VI Ref"=w414, "Playback in"=w418) -> ("Playback out"=w415:refnum<vi>)  [unwired: 8 in]
            n258 = register-events(w415) -> (reference out=w417:refnum<event-registration>, error out=w416:errorcluster)  [unwired: 2 in]
          }
        }
        n259 = global write "WPI_DashboardLogging Global.vi" "Recording"(w408) -> ()
        n260 = property on="Camera Image" class="ImageControl"("Image Information Shown"=w400, "Image Information Visible"=w399) -> ()  [unwired: 2 in, 2 out]
        n261 = call <vilib>:"WPI_DashboardNT Log FieldName Cache.vi"("Operation"=enum16{"Lookup/Add", "Index", "Clear"}."Clear") -> ()  [unwired: 8 in, 3 out]
      }
      event Panel Close {
        w419 = enum32{"Stop", "Record", "Playback"}."Stop" ("Rec Mode")
        n262 = event-data() -> ()  [unwired: 1 in, 4 out]
        n263 = local write "Rec Mode"(w419) -> ()
        n264 = global write "WPI_DashboardLogging Global.vi" "Recording"(w419) -> ()
      }
      event Panel Close {
        # "Abort playback window and ourself"
        n265 = event-data() -> ()  [unwired: 1 in, 4 out]
        n266 = invoke class="VI" method="FP.Close"(reference=w424) -> (reference out=w423:refnum<vi>)  [unwired: 2 in, 2 out]
        n267 = invoke class="VI" method="Abort VI"(reference=w423) -> (error out=w422:errorcluster)  [unwired: 2 in, 2 out]
        n268 = invoke class="VI" method="Abort VI"(error in=w422) -> ()  [unwired: 2 in, 3 out]
      }
    }
  }
  n269 = property on="On/Off" class="Bool (strict)"("Visible"=w25) -> ()  [unwired: 2 in, 2 out]
  n270 = property on="Motor" class="Clust (strict)"("Visible"=w25) -> ()  [unwired: 2 in, 2 out]
  n271 = property on="Progress" class="Clust (strict)"("Visible"=w25) -> ()  [unwired: 2 in, 2 out]
  n272 = property on="Test Ring" class="Ring (strict)"("Visible"=w25) -> ()  [unwired: 2 in, 2 out]
  n273 = property on="Rev/Fwd" class="Clust (strict)"("Visible"=w25) -> ()  [unwired: 2 in, 2 out]
  n274 = property on="Camera Settings" class="Clust (strict)"("Visible"=w25) -> ()  [unwired: 2 in, 2 out]
  n275 = local write "DB Camera Config"(w25) -> ()
  n276 = global write "WPI_DashboardLogging Global.vi" "Recording"(w8) -> ()
  n277 = local write "Rec Mode"(w8) -> ()
